vi "autolock2.vi"(9 "Cluster":T1, 10 "Mid":bool, 11 "Top":bool) -> (3 "S_top":dbl)   [LabVIEW 2012]
uses:
  <vilib>/Rock Robotics/WPI/RobotDrive/WPI_RobotDriveGetSetRefNum.vi
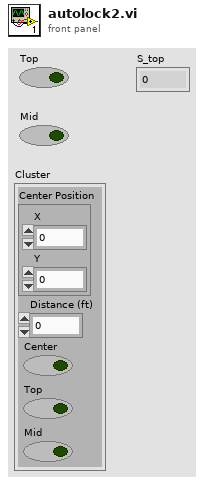
[diagram p1: front panel]
types:
  T1 = cluster{"Center Position":cluster{"X":dbl, "Y":dbl}, "Distance (ft)":dbl, "Center":bool, "Top":bool, "Mid":bool}
  T2 = typedef "WPI_RobotDriveDevRef.ctl" = cluster{"DevStatus":errorcluster, "Motors[]":T3[], "Square Inputs":bool, "Max Output":dbl, "Isochronous":bool}
  T3 = typedef "WPI_MotorControlDeviceRef.ctl" = cluster{"DeviceStatus":errorcluster, "Type":enum16{"PWM", "CAN"}, "PWM":cluster{"Digital Module":T4, "PWM Channel":T5, "DeadBand":T6}, "CAN":cluster{"Device Number":u8, "Control Mode":T7, "Semaphore":T8, "Max Vout":dbl}, "Invert":bool, "TransformRef":T9, "InvTransformRef":T9}
  T4 = typedef "FPGA_TypedefDigitalModule.ctl" = enum16{"Digital Module 1", "Digital Module 2"}
  T5 = typedef "FPGA_DIOPWMChannel.ctl" = enum8{"PWM 1", "PWM 2", "PWM 3", "PWM 4", "PWM 5", "PWM 6", "PWM 7", "PWM 8", "PWM 9", "PWM 10", "Invalid"}
  T6 = typedef "WPI_PWMDeadband.ctl" = cluster{"Name":string, "maxPositivePwm":i32, "minPositivePwm":i32, "centerPwm":i32, "maxNegativePwm":i32, "minNegativePwm":i32, "angularRange":u16}
  T7 = typedef "WPI_CANJaguar_ControlMode.ctl" = enum8{"Percent VBus", "Current", "Speed", "Position", "Voltage"}
  T8 = typedef "Semaphore RefNum" = refnum<k1>
  T9 = typedef "WPI_PWMTransform_ConPane.ctl" = refnum<vi>
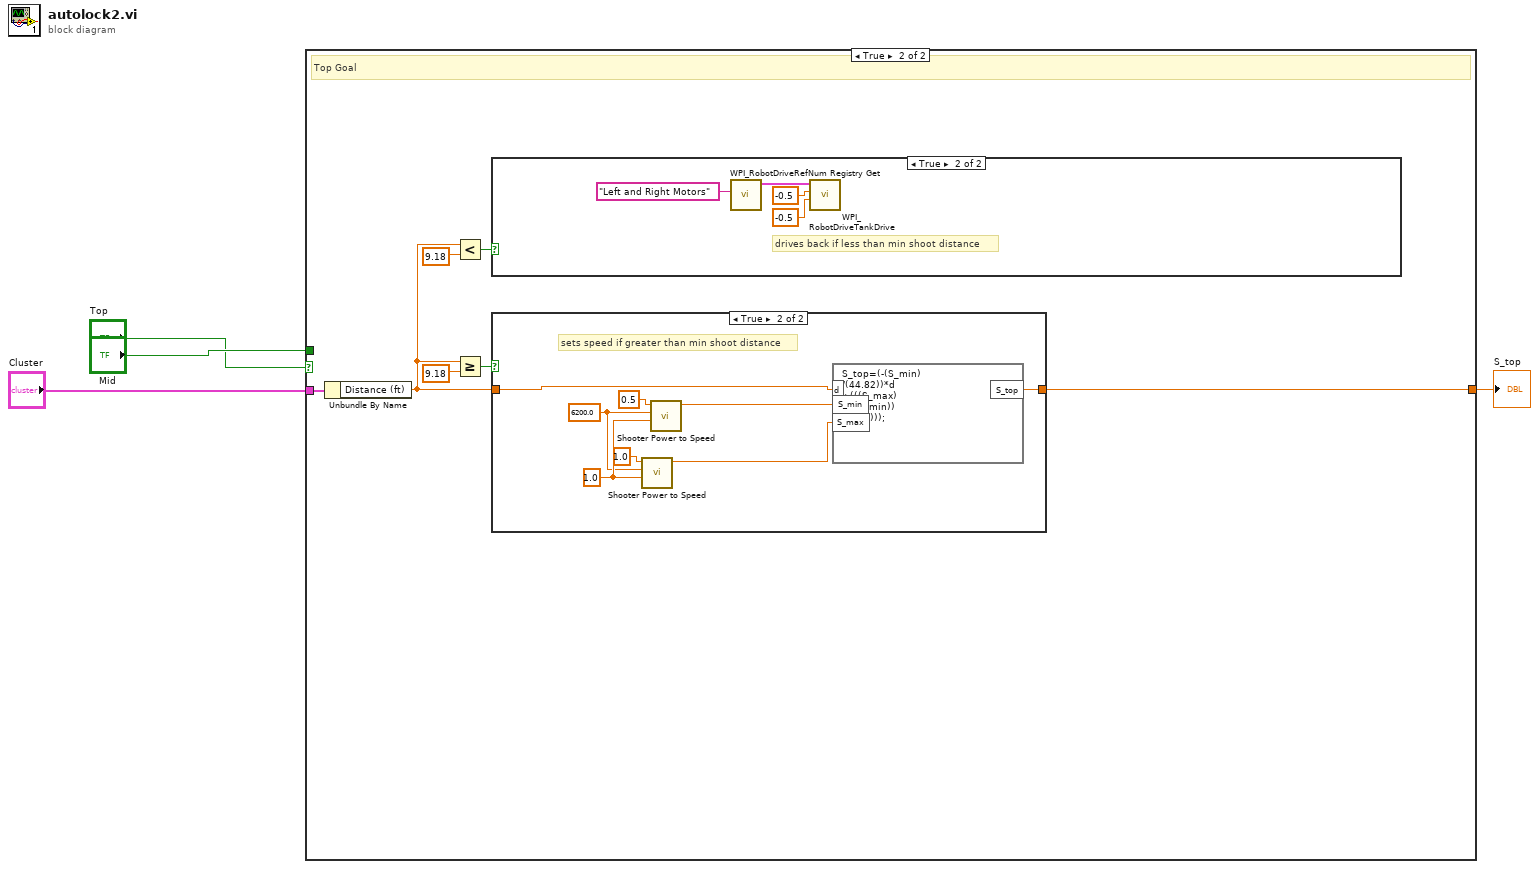
[diagram p0: block diagram]
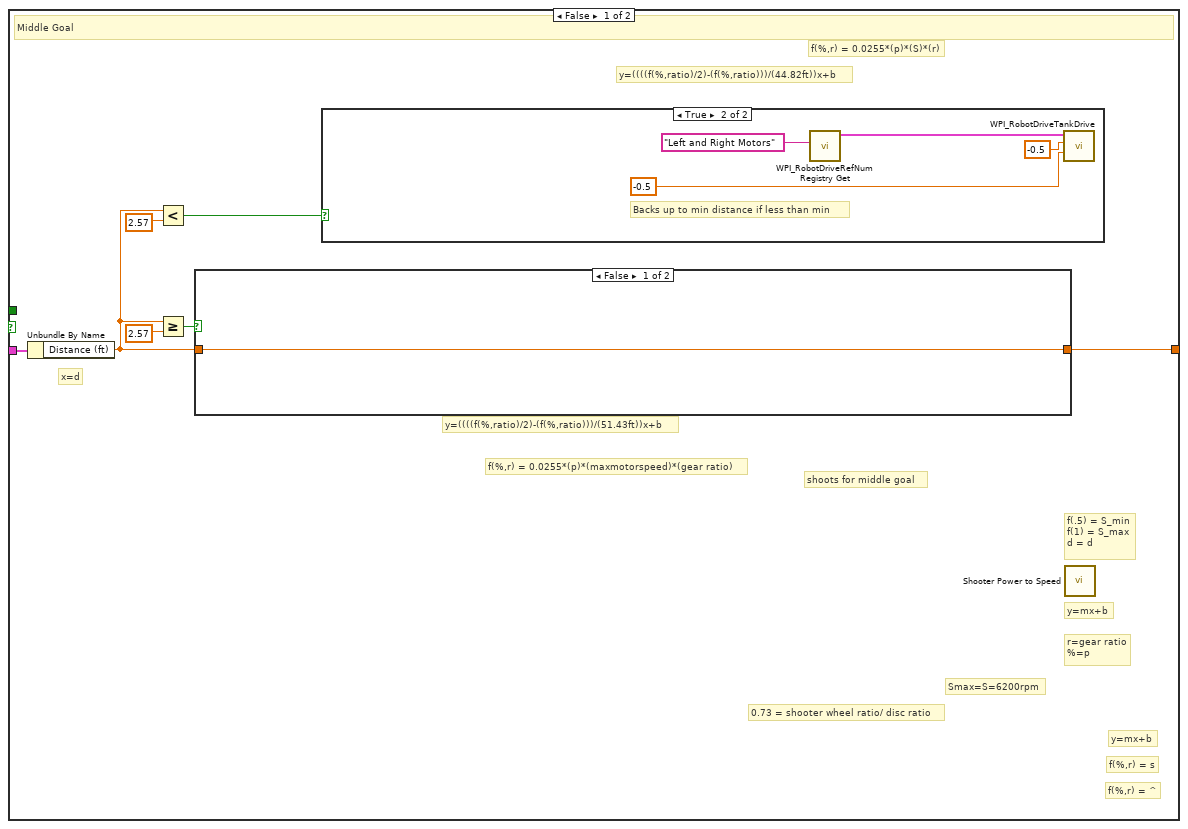
[diagram p2: hidden frame]
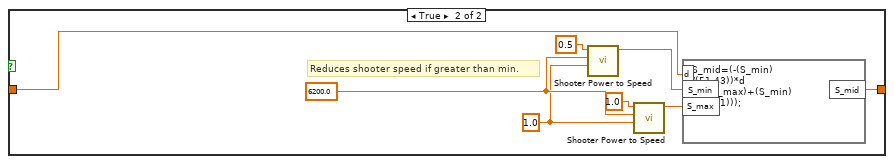
[diagram p4: hidden frame]
diagram:
  n1 = case shown="True" "Top" {
    tunnel: "Cluster" -> [w11 w31]
    tunnel: [w5 w25] -> w2
    tunnel: "Mid" -> [_ _]
    frame False {
      # "f(.5) = S_min\nf(1) = S_max\nd = d"
      # "y=mx+b"
      # "0.73 = shooter wheel ratio/ disc ratio"
      # "f(%,r) = ^"
      # "x=d"
      # "y=mx+b"
      # "Smax=S=6200rpm"
      # "f(%,r) = 0.0255*(p)*(S)*(r)"
      # "f(%,r) = 0.0255*(p)*(maxmotorspeed)*(gear ratio)"
      # "r=gear ratio\n%=p"
      # "y=((((f(%,ratio)/2)-(f(%,ratio)))/(51.43ft))x+b"
      # "f(%,r) = s"
      # "y=((((f(%,ratio)/2)-(f(%,ratio)))/(44.82ft))x+b"
      # "shoots for middle goal"
      # "Middle Goal"
      n2 = Unbundle By Name(w11) -> ("Distance (ft)"=w6:dbl)
      n3 = Less?(x=w6, y=2.57) -> (x < y?=w8:bool)
      n4 = Greater Or Equal?(x=w6, y=2.57) -> (x >= y?=w7:bool)
      n5 = case shown="False" w7 {
        tunnel: w6 -> [w16 w19]
        tunnel: [w16 w20] -> w5
        frame False {
        }
        frame True {
          w23 = 6200.0 ("Shooter Maxiimum Speed (rpm)")
          w22 = 1.0 ("Shooter Wheel/Gear Ratio")
          # "Reduces shooter speed if greater than min."
          n6 = call "Shooter Power to Speed.vi"("Shooter Wheel/Gear Ratio"=w22, "Shooter Maxiimum Speed (rpm)"=w23, "Shooter Power (%)"=0.5) -> ("Disc Speed"=w17:dbl)  [unwired: 8 in]
          n7 = call "Shooter Power to Speed.vi"("Shooter Wheel/Gear Ratio"=w22, "Shooter Maxiimum Speed (rpm)"=w23, "Shooter Power (%)"=1.0) -> ("Disc Speed"=w18:dbl)  [unwired: 8 in]
          n8 = formula code="S_mid=(-(S_min)\n/(51.43))*d\n+(((S_max)+(S_min)\n/(20.01)));"("d"=w19, "S_min"=w17, "S_max"=w18) -> ("S_mid"=w20:dbl)
        }
      }
      n9 = case shown="True" w8 {
        frame False {
        }
        frame True {
          # "Backs up to min distance if less than min"
          n10 = call <vilib>:"WPI_RobotDriveRefNum Registry Get.vi"("refnum name"="Left and Right Motors") -> ("RobotDriveDevRef"=w13:T2)  [unwired: 9 in, 1 out]
          n11 = call <vilib>:"WPI_RobotDriveTankDrive.vi"("Right axis value"=-0.5, "Left axis value"=-0.5, "RobotDriveDevRef"=w13) -> ()  [unwired: 6 in, 3 out]
        }
      }
      n12 = call "Shooter Power to Speed.vi"() -> ()  [unwired: 11 in, 1 out]
    }
    frame True {
      # "Top Goal"
      n13 = Unbundle By Name(w31) -> ("Distance (ft)"=w26:dbl)
      n14 = Less?(x=w26, y=9.18) -> (x < y?=w27:bool)
      n15 = Greater Or Equal?(x=w26, y=9.18) -> (x >= y?=w30:bool)
      n16 = case shown="True" w27 {
        frame False {
        }
        frame True {
          # "drives back if less than min shoot distance"
          n17 = call <vilib>:"WPI_RobotDriveRefNum Registry Get.vi"("refnum name"="Left and Right Motors") -> ("RobotDriveDevRef"=w32:T2)  [unwired: 1 in, 9 out]
          n18 = call <vilib>:"WPI_RobotDriveTankDrive.vi"("Right axis value"=-0.5, "Left axis value"=-0.5, "RobotDriveDevRef"=w32) -> ()  [unwired: 6 in, 3 out]
        }
      }
      n19 = case shown="True" w30 {
        tunnel: w26 -> [w36 w39]
        tunnel: [w36 w40] -> w25
        frame False {
        }
        frame True {
          w42 = 6200.0 ("Shooter Maxiimum Speed (rpm)")
          w43 = 1.0 ("Shooter Wheel/Gear Ratio")
          # "sets speed if greater than min shoot distance"
          n20 = call "Shooter Power to Speed.vi"("Shooter Wheel/Gear Ratio"=w43, "Shooter Maxiimum Speed (rpm)"=w42, "Shooter Power (%)"=1.0) -> ("Disc Speed"=w37:dbl)  [unwired: 8 in]
          n21 = call "Shooter Power to Speed.vi"("Shooter Wheel/Gear Ratio"=w43, "Shooter Maxiimum Speed (rpm)"=w42, "Shooter Power (%)"=0.5) -> ("Disc Speed"=w44:dbl)  [unwired: 8 in]
          n22 = formula code="S_top=(-(S_min)\n/(44.82))*d\n+(((S_max)\n+((S_min))\n/(4.88)));"("d"=w39, "S_min"=w44, "S_max"=w37) -> ("S_top"=w40:dbl)
        }
      }
    }
  }
  "S_top" <- w2
